vi "FGV Dewar Befuellung.vi"(0 "Aktion":T1, 11 "error in (no error)":errorcluster caption="Fehler (Eingang, kein Fehler)") -> (4 "Befüllung":bool, 15 "error out":errorcluster caption="Fehler (Ausgang)")   [LabVIEW 2020, in "Stickstoff Befuellung.lvlib"]
uses:
  Stickstoff Befuellung.lvlib
  Aktion FGV Dewar Befuellung.ctl
  Verwaltung/FGV OUT Aktionen.ctl
  Verwaltung/FGV IN Aktionen.ctl
  Verwaltung/Verwaltung - cRIO.lvlib
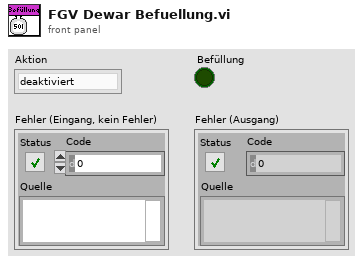
[diagram p1: front panel]
types:
  T1 = typedef "Stickstoff Befuellung.lvlib/Aktion FGV Dewar Befuellung.ctl" = enum16{"deaktiviert", "Befüllung aktiv", "prüfen"}
  T2 = typedef "Verwaltung - cRIO.lvlib/FGV OUT Aktionen.ctl" = enum16{"lesen", "ANA OUT", "DO 0-31", "DO 32-47"}
  T3 = typedef "Verwaltung - cRIO.lvlib/FGV IN Aktionen.ctl" = enum16{"lesen", "DI", "AI", "Fühler Br.", "TC", "Fühler Br. TC"}
  T4 = typedef "Verwaltung - cRIO.lvlib/Digital Ausgaenge 32-63.ctl" = cluster{"O32: Messgaspumpe EIN":bool, "O33: (Umgebungsluftpumpe)":bool, "O34: (Kondensatpumpe GK)":bool, "O35: Klima/Lüfter EIN":bool, "O36: Versorgung Heizungen":bool, "O37: Versorgung Heizungen":bool, "O38: (Gaskühler EIN (Freigabe))":bool, "O39: Störung FAS LP":bool, "O40: (Heizung Filterblock)":bool, "O41: Heizung HL zu FT-IR":bool, "O42: Heizung HL Extern SP1":bool, "O43: Heizung HL Extern SP2":bool, "O44: Heizung Reserve":bool, "O45: Heizung Reserve":bool, "O46: Statusbeleuchtung grün":bool, "O47: (Statusbeleuchtung rot) Dewar Extern N2 Einblasung":bool}
  T5 = typedef "Verwaltung - cRIO.lvlib/Digital Eingaenge 0-15.ctl" = cluster{"I0: N2 Nachf. FT-IR voll":bool, "I1: N2 Nachf. Vorrat leer":bool, "I2: (Klimaanlage eingeschaltet)":bool, "I3: (Klimaanlage Störung)":bool, "I4: Trigger Eingang (Messdaten sp.)":bool, "I5: Reserve":bool, "I6: 50l Dewar angeschlossen":bool, "I7: Reserve":bool, "I8: Druckschalter Versorgung ok":bool, "I9: N2 Nachf. Vorrat voll":bool, "I10: N2 50l Vorrat leer":bool, "I11: Reserve":bool, "I12: Drucksch. N2 Versorgung":bool, "I13: Reserve":bool, "I14: Reserve":bool, "I15: (Füllstand Kondensatbehälter)":bool}
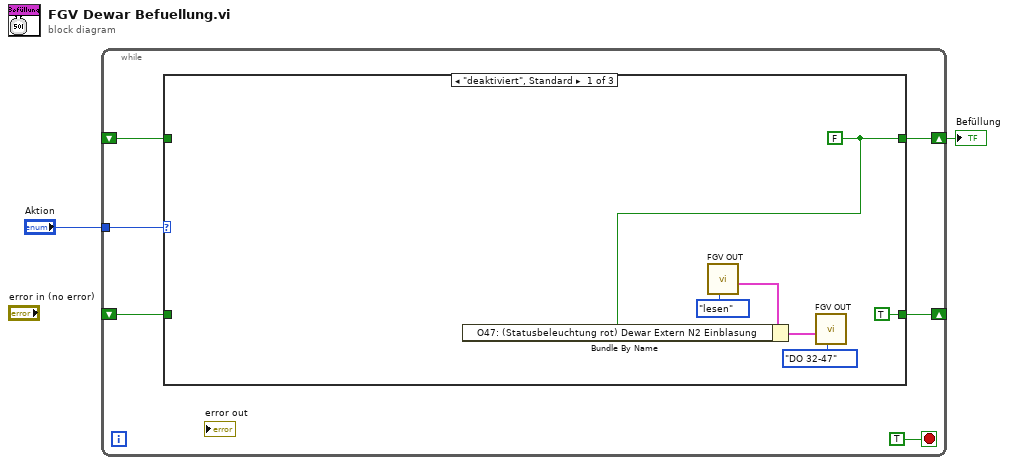
[diagram p0: block diagram]
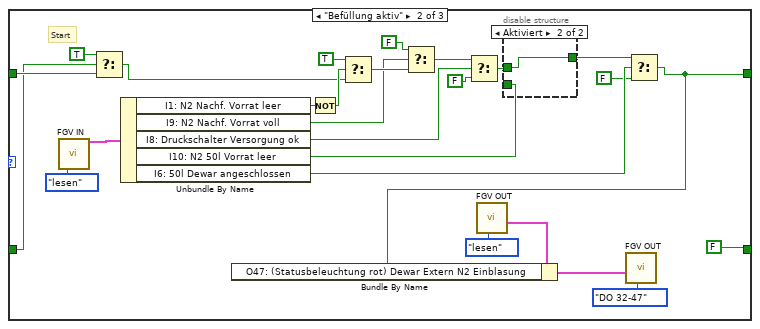
[diagram p2: hidden frame]
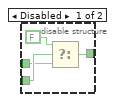
[diagram p3: hidden frame]
diagram:
  n1 = while {
    shift-right: [w7] -> w1
    shift-left: _ -> [w6]
    tunnel: "Aktion" -> [w5]
    shift-right: [w4] -> _
    shift-left: _ -> [w3]
    stop <- TRUE stop-if-true
    n2 = case shown="\"deaktiviert\", Standard" w5 {
      tunnel: [w9 w15 w47] -> w7
      tunnel: w6 -> [_ w23 w47]
      tunnel: [TRUE ("t") FALSE ("t") w46] -> w4
      tunnel: w3 -> [_ w20 w46]
      frame "deaktiviert", Default {
        w9 = FALSE
        n3 = call "FGV OUT.vi"("Aktion"=FGV_OUT_Aktionen."lesen") -> ("DO 32-63"=w12:T4)  [unwired: 7 in, 3 out]
        n4 = Bundle By Name(cluster=w12, "O47: (Statusbeleuchtung rot) Dewar Extern N2 Einblasung"=w9) -> (w10:T4)
        n5 = call "FGV OUT.vi"("Aktion"=FGV_OUT_Aktionen."DO 32-47", "DO 32-63"=w10) -> ()  [unwired: 6 in, 4 out]
      }
      frame "Befüllung aktiv" {
        # "Start"
        n6 = call "FGV IN.vi"("Aktion"=FGV_IN_Aktionen."lesen") -> ("DI"=w40:T5)  [unwired: 10 in, 4 out]
        n7 = Select(t=TRUE, s=w20, f=w23) -> (s? t:f=w22:bool)
        n8 = Unbundle By Name(w40) -> ("I1: N2 Nachf. Vorrat leer"=w38:bool, "I9: N2 Nachf. Vorrat voll"=w35:bool, "I8: Druckschalter Versorgung ok"=w33:bool, "I10: N2 50l Vorrat leer"=w30:bool, "I6: 50l Dewar angeschlossen"=w28:bool)
        n9 = Not(x=w38) -> (.not. x?=w25:bool)
        n10 = Select(t=TRUE, s=w25, f=w22) -> (s? t:f=w36:bool)
        n11 = Select(t=FALSE, s=w35, f=w36) -> (s? t:f=w32:bool)
        n12 = Select(t=w32, s=w33, f=FALSE) -> (s? t:f=w29:bool)
        n13 = call "FGV OUT.vi"("Aktion"=FGV_OUT_Aktionen."lesen") -> ("DO 32-63"=w18:T4)  [unwired: 7 in, 3 out]
        n14 = disable-structure shown="Aktiviert" {
          disable-tunnel: w30 -> [w44 _]
          disable-tunnel: w29 -> [w42 w45]
          disable-tunnel: [w41 w45] -> w26
          frame Disabled {
            n15 = Select(t=FALSE ("f"), s=w44, f=w42) -> (s? t:f=w41:bool)
          }
          frame Enabled {
          }
        }
        n16 = Select(t=w26, s=w28, f=FALSE) -> (s? t:f=w15:bool)
        n17 = Bundle By Name(cluster=w18, "O47: (Statusbeleuchtung rot) Dewar Extern N2 Einblasung"=w15) -> (w16:T4)
        n18 = call "FGV OUT.vi"("Aktion"=FGV_OUT_Aktionen."DO 32-47", "DO 32-63"=w16) -> ()  [unwired: 6 in, 4 out]
      }
      frame "prüfen" {
      }
    }
  }
  "Befüllung" <- w1
